vi "Name Formatter Main.vi"(1 "Case Type":T1, 2 "Input string":string) -> (7 "Output string":string)   [LabVIEW 2025, in "Name Formatter.lvlib"]
doc: "Description:\nThe <b>MainModule</b> acts as the entry point. It receives a text with words separated by spaces and delegates the conversion to one of the available formatting modules: <b>Spaced Camel Case</b>, <b>camelCase</b>, <b>PascalCase</b>, <b>snake_case</b>, or <b>kebab-case</b>.\n\nExample:\nInput -> hello cruel world(selected: <b>PascalCase</b>)\nOutput -> HelloCruelWorld\n\nRequirements:\nThe input must contain spaces. Without spaces, this conversion cannot be applied."
uses:
  Name Formatter.lvlib
  Case Type--enum.ctl
panel:
  # "string with spaces"
  # "formatted string"
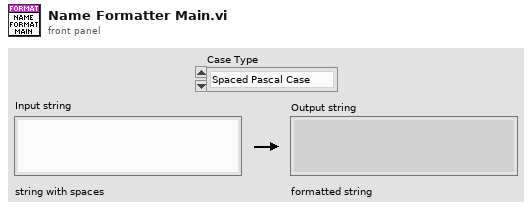
[diagram p1: front panel]
types:
  T1 = typedef "Name Formatter.lvlib/Case Type--enum.ctl" = enum16{"Spaced Pascal Case", "camelCase", "PascalCase", "snake_case", "kebab-case"}
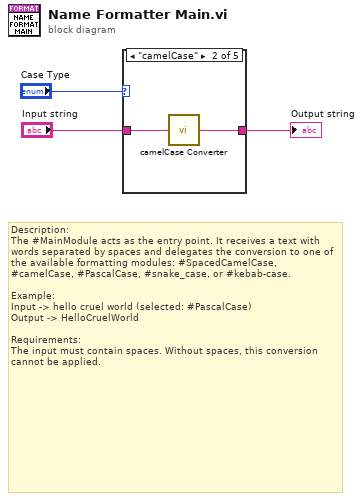
[diagram p0: block diagram]
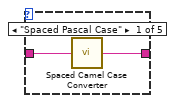
[diagram p2: hidden frame]
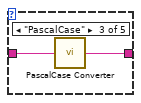
[diagram p3: hidden frame]
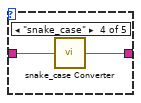
[diagram p4: hidden frame]
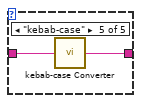
[diagram p5: hidden frame]
diagram:
  # "Description:\nThe #MainModule acts as the entry point. It receives a text with words separated by spaces and delegates the conversion to one of the available formatting modules: #SpacedCamelCase, #camelCase, #PascalCase, #snake_case, or #kebab-case.\n\nExample:\nInput -> hello cruel world (selected: #PascalCase)\nOutput -> HelloCruelWorld\n\nRequirements:\nThe input must contain spaces. Without spaces, this conversion cannot be applied."
  n1 = case shown="\"camelCase\"" "Case Type" {
    tunnel: "Input string" -> [w5 w7 w9 w11 w13]
    tunnel: [w4 w6 w8 w10 w12] -> w2
    frame "Spaced Pascal Case" {
      n2 = call "Spaced Camel Case Converter.vi"("Input string"=w5) -> ("Output string"=w4:string)  [unwired: 4 in]
    }
    frame "camelCase" {
      n3 = call "camelCase Converter.vi"("Input string"=w7) -> ("Output string"=w6:string)  [unwired: 4 in]
    }
    frame "PascalCase" {
      n4 = call "PascalCase Converter.vi"("Input string"=w9) -> ("Output string"=w8:string)  [unwired: 4 in]
    }
    frame "snake_case" {
      n5 = call "snake_case Converter.vi"("Input string"=w11) -> ("Output string"=w10:string)  [unwired: 4 in]
    }
    frame "kebab-case" {
      n6 = call "kebab-case Converter.vi"("Input string"=w13) -> ("Output string"=w12:string)  [unwired: 4 in]
    }
  }
  "Output string" <- w2
